vi "Close.vi"(8 "error in (no error)":errorcluster, 11 "SigGen_MXG in":refnum<class "SigGen_MXG.lvclass">) -> (0 "error out":errorcluster)   [LabVIEW 2014, in "SigGen_MXG.lvclass"]
uses:
  SigGen_MXG.lvclass
  SigGen_MXG.lvclass/SigGen_MXG.ctl
  data/Agilent PSG MXG Series.lvlib
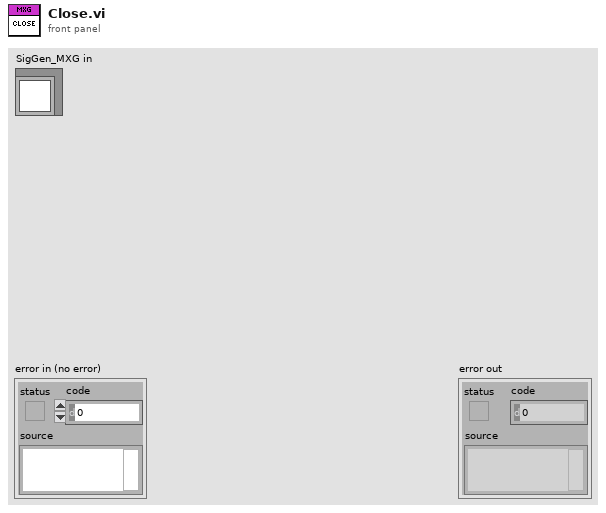
[diagram p1: front panel]
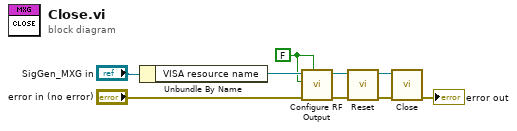
[diagram p0: block diagram]
diagram:
  w1 = FALSE ("Enable Modulation (T:Enable)")
  n1 = Unbundle By Name("SigGen_MXG in") -> ("VISA resource name"=w9:refnum<visa-resource-name>)
  n2 = call "Configure RF Output.vi"("Enable Modulation (T:Enable)"=w1, "error in (no error)"="error in (no error)", "Enable RF Output (F:Disable)"=w1, "VISA resource name"=w9) -> ("error out"=w3:errorcluster, "VISA resource name out"=w5:refnum<visa-resource-name>)  [unwired: 4 in, 2 out]
  n3 = call "Reset.vi"("error in (no error)"=w3, "VISA resource name"=w5) -> ("error out"=w2:errorcluster, "VISA resource name out"=w4:refnum<visa-resource-name>)  [unwired: 8 in]
  n4 = call "Close.vi"("error in (no error)"=w2, "VISA resource name"=w4) -> ("error out"=→"error out":errorcluster)  [unwired: 9 out]
